vi "Convert_Distance_to_Flywheel_Velocity.vi"(9 "angle":dbl, 10 "distance":dbl, 11 "terminal height":dbl=90.5) -> (3 "velocity":dbl)   [LabVIEW 2019]
panel:
  in  "wheel diameter":dbl=4.0
  in  "ball diameter":dbl=7.0
  in  "initial height":dbl=25.0
  in  "gear ratio":dbl=1.0
  in  "compression":dbl=2.25
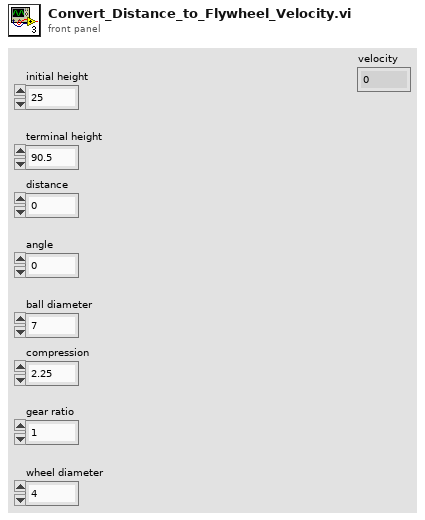
[diagram p1: front panel]
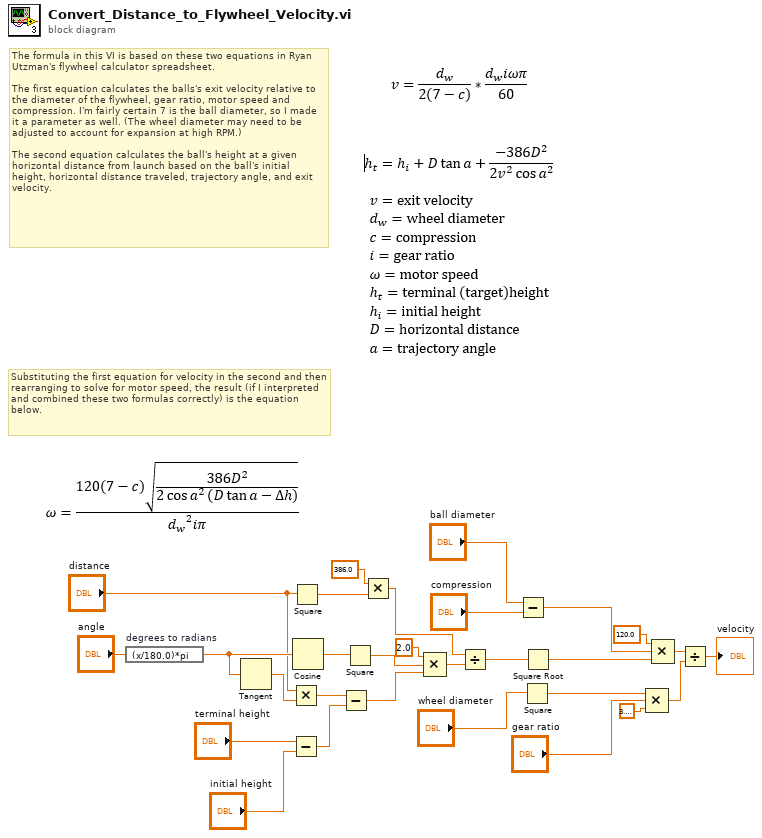
[diagram p0: block diagram]
diagram:
  # "Substituting the first equation for velocity in the second and then rearranging to solve for motor speed, the result (if I interpreted and combined these two formulas correctly) is the equation below."
  # "The formula in this VI is based on these two equations in Ryan Utzman's flywheel calculator spreadsheet.\n\nThe first equation calculates the balls's exit velocity relative to the diameter of the flywheel, gear ratio, motor speed and compression. I'm fairly certain 7 is the ball diameter, so I made it a parameter as well. (The wheel diameter may need to be adjusted to account for expansion at high RPM.)\n\nThe second equation calculates the ball's height at a given horizontal distance from launch based on the ball's initial height, horizontal distance traveled, trajectory angle, and exit velocity."
  n1 = expression code="(x/180.0)*pi" "degrees to radians"("angle") -> (w28:dbl)
  n2 = Tangent(1:w28) -> (0:w20:dbl)
  n3 = Multiply(x="distance", y=w20) -> (x*y=w19:dbl)
  n4 = Subtract(x="terminal height", y="initial height") -> (x-y=w18:dbl)
  n5 = Square(x="distance") -> (x^2=w25:dbl)
  n6 = Cosine(x=w28) -> (cos(x)=w22:dbl)
  n7 = Subtract(x=w19, y=w18) -> (x-y=w17:dbl)
  n8 = Square(x=w22) -> (x^2=w21:dbl)
  n9 = Multiply(x=386.0, y=w25) -> (x*y=w16:dbl)
  n10 = Compound Arithmetic op=MULTIPLY(2.0 ("value"), w21, w17) -> (w15:dbl)
  n11 = Divide(x=w16, y=w15) -> (x/y=w11:dbl)
  n12 = Subtract(x="ball diameter", y="compression") -> (x-y=w2:dbl)
  n13 = Square(x="wheel diameter") -> (x^2=w9:dbl)
  n14 = Square Root(x=w11) -> (sqrt(x)=w1:dbl)
  n15 = Compound Arithmetic op=MULTIPLY(w9, "gear ratio", 3.141592653589793) -> (w5:dbl)
  n16 = Compound Arithmetic op=MULTIPLY(120.0 ("value"), w2, w1) -> (w6:dbl)
  n17 = Divide(x=w6, y=w5) -> (x/y=→"velocity":dbl)
